vi "Draw Filled Rect.vi"(8 "Limits":dbl[](array[numeric]), 9 "Scores":dbl[](array[numeric]), 10 "Bounding Box":T2, 11 "image in":T1) -> (3 "image out":T1)   [LabVIEW 2012]
doc: "Add a rectangle border around the inside and outside of what is believed to be the reflective tape. Also place the color coded scores next to all of the large blobs being processed."
uses:
  <vilib>/vision/Image Controls.llb/IMAQ Image.ctl
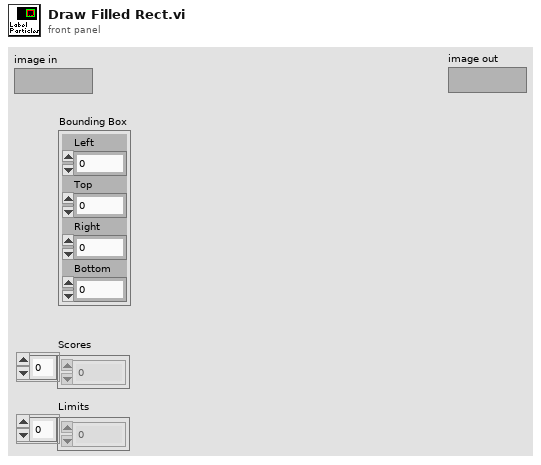
[diagram p1: front panel]
types:
  T1 = typedef "IMAQ Image.ctl" = refnum<image>
  T2 = cluster{"Left":dbl, "Top":dbl, "Right":dbl, "Bottom":dbl}
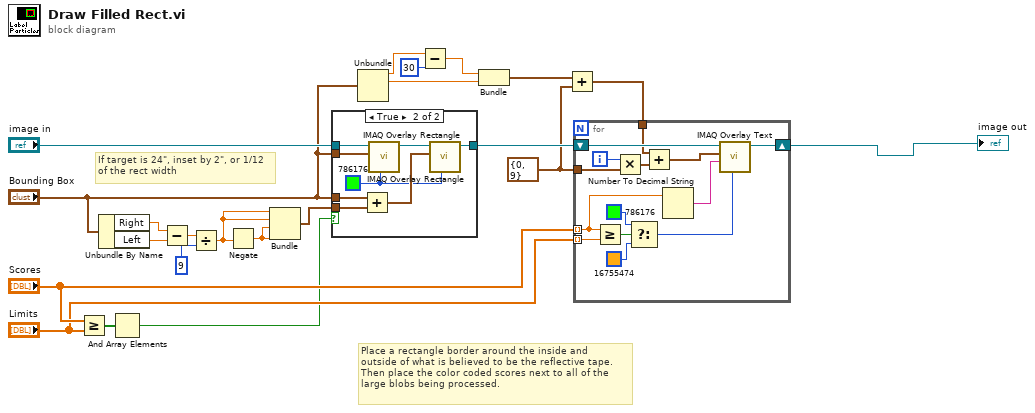
[diagram p0: block diagram]
diagram:
  w9 = cluster{i32, i32} {0, 9}
  # "Place a rectangle border around the inside and\noutside of what is believed to be the reflective tape.\nThen place the color coded scores next to all of the\nlarge blobs being processed."
  # "If target is 24\", inset by 2\", or 1/12\nof the rect width"
  n1 = Greater Or Equal?(x="Scores", y="Limits") -> (x >= y?=w21:bool[])
  n2 = Unbundle By Name("Bounding Box") -> ("Right"=w7:dbl, "Left"=w6:dbl)
  n3 = And Array Elements(Boolean array=w21) -> (logical AND=w18:bool)
  n4 = Subtract(x=w7, y=w6) -> (x-y=w4:dbl)
  n5 = Divide(x=w4, y=9) -> (x/y=w2:dbl)
  n6 = Negate(x=w2) -> (-x=w8:dbl)
  n7 = Bundle(w2, w2, w8, w8) -> (w5:cluster{dbl, dbl, dbl, dbl})  [unwired: 1 in]
  n8 = case shown="True" w18 {
    tunnel: "image in" -> [w23 w31]
    tunnel: "Bounding Box" -> [_ w30]
    tunnel: "Bounding Box" -> [_ w28]
    tunnel: [w23 w26] -> w16
    tunnel: w5 -> [_ w24]
    frame False {
    }
    frame True {
      w25 = u32 786176 ("Color")
      n9 = Add(x=w28, y=w24) -> (x+y=w27:cluster{dbl, dbl, dbl, dbl})
      n10 = call "IMAQ Overlay Rectangle"("Color"=w25, "Rectangle"=w30, "Image"=w31) -> ("Image Out"=w29:T1)  [unwired: 3 in, 5 out]
      n11 = call "IMAQ Overlay Rectangle"("Color"=w25, "Rectangle"=w27, "Image"=w29) -> ("Image Out"=w26:T1)  [unwired: 3 in, 5 out]
    }
  }
  n12 = Unbundle("Bounding Box") -> ("Left"=w14:dbl, "Top"=w15:dbl)  [unwired: 2 out]
  n13 = Subtract(x=w14, y=30) -> (x-y=w13:dbl)
  n14 = Bundle(w13, "Top"=w15) -> (w11:cluster{dbl, "Top":dbl})  [unwired: 1 in]
  n15 = Add(x=w11, y=w9) -> (x+y=w10:cluster{dbl, dbl})
  n16 = for {
    shift-right: [w44] -> w1
    shift-left: w16 -> [w45]
    tunnel: "Scores" -> [w37] mode=indexing
    tunnel: "Limits" -> [w43] mode=indexing
    tunnel: w9 -> [w34]
    tunnel: w10 -> [w33]
    i -> [w36]
    n17 = Greater Or Equal?(x=w37, y=w43) -> (x >= y?=w42:bool)
    n18 = Multiply(x=w36, y=w34) -> (x*y=w35:cluster{i32, i32})
    n19 = Select(t=u32 786176 ("Color"), s=w42, f=u32 16755474 ("Color")) -> (s? t:f=w38:u32)
    n20 = Add(x=w33, y=w35) -> (x+y=w32:cluster{dbl, dbl})
    n21 = Number To Decimal String(number=w37) -> (decimal integer string=w39:string)  [unwired: 1 in]
    n22 = call "IMAQ Overlay Text"("Text Color (black)"=w38, "String"=w39, "Origin"=w32, "Image"=w45) -> ("Image Out"=w44:T1)  [unwired: 6 in, 1 out]
  }
  "image out" <- w1
